vi "DriveExecute_StateSpaceCtrl_1.vi"(8 "error in (no error)":errorcluster) -> (0 "error out":errorcluster)   [LabVIEW 2020]
doc: "Execute for Drie\n\nClosed control loop for drive\n\ninput: \n error in (cluster)\n\noutput:\n error out (cluster)"
uses:
  <vilib>/Rock Robotics/WPI/ThirdParty/Phoenix-LabVIEW/Motor Controller/Controls/CTRE_Phoenix_MotorControl_ControlMode.ctl
  <vilib>/Rock Robotics/WPI/ThirdParty/JAS_Junk/TrajLib/SimpleMotorFF_Calculate.vi
  <vilib>/Rock Robotics/WPI/ThirdParty/JAS_Junk/TrajLib/VI/Util_GetTime_U32.vi
  <vilib>/Rock Robotics/WPI/ThirdParty/JAS_Junk/TrajLib/PIDController_AtSetpoint.vi
  <vilib>/Rock Robotics/WPI/ThirdParty/JAS_Junk/TrajLib/PIDController_SetPIDF.vi
  <vilib>/Rock Robotics/WPI/ThirdParty/JAS_Junk/TrajLib/PIDController_SetDerivativeFilter.vi
  <vilib>/Rock Robotics/WPI/ThirdParty/JAS_Junk/TrajLib/PIDController_SetIntegratorRange.vi
  <vilib>/Rock Robotics/WPI/ThirdParty/JAS_Junk/TrajLib/PIDController_SetTolerancePandV.vi
  <vilib>/Rock Robotics/WPI/ThirdParty/JAS_Junk/TrajLib/PIDController_DisableContinousInput.vi
  <vilib>/Rock Robotics/WPI/ThirdParty/JAS_Junk/TrajLib/PIDController_EnableContinousInput.vi
  <vilib>/Rock Robotics/WPI/ThirdParty/JAS_Junk/TrajLib/PIDController_Reset.vi
  <vilib>/Rock Robotics/WPI/ThirdParty/JAS_Junk/TrajLib/PIDController_New.vi
  <vilib>/Rock Robotics/WPI/ThirdParty/JAS_Junk/TrajLib/PIDController_SetOutputLimits.vi
  <vilib>/Rock Robotics/WPI/ThirdParty/JAS_Junk/TrajLib/SlewRateLimiter_New.vi
  <vilib>/Rock Robotics/WPI/ThirdParty/JAS_Junk/TrajLib/SlewRateLimiter_Reset.vi
  <vilib>/Rock Robotics/WPI/ThirdParty/JAS_Junk/TrajLib/SlewRateLimiter_Calculate.vi
  <vilib>/Rock Robotics/WPI/ThirdParty/JAS_Junk/TrajLib/SlewRateLimiter_SetRate.vi
  <vilib>/Rock Robotics/WPI/ThirdParty/JAS_Junk/TrajLib/PIDController_NewPeriod.vi
  <vilib>/Rock Robotics/SystemInterfaces/NetworkCommunication/NetComm_UsageReport_report.vi
  <vilib>/Rock Robotics/SystemInterfaces/Utilities/FPGA_UtilitiesRead LocalTime.vi
  <vilib>/Rock Robotics/WPI/ThirdParty/JAS_Junk/TrajLib/VI/Util_GetTime_U64.vi
  DriveGlobal.vi
  <vilib>/Rock Robotics/WPI/ThirdParty/Phoenix-LabVIEW/Motor Controller/Get/CTRE_Phoenix_MotorController_GetSelectedSensorData.vi
  <vilib>/Rock Robotics/WPI/ThirdParty/JAS_Junk/TrajLib/Globals/Util_LibraryGlobals.vi
  <vilib>/Rock Robotics/WPI/ThirdParty/JAS_Junk/TrajLib/PIDController_AdvCalculate_FF_Sp_Pv.vi
  <vilib>/Rock Robotics/WPI/ThirdParty/JAS_Junk/TrajLib/Trajectory_Library.lvlib
  <vilib>/Rock Robotics/WPI/ThirdParty/JAS_Junk/TrajLib/Enum/DCMOTOR_TYPES_ENUM.ctl
  <vilib>/Rock Robotics/WPI/ThirdParty/JAS_Junk/TrajLib/Enum/DIFF_DRIVE_ToughBoxMini_GearChoice_ENUM.ctl
  <vilib>/Rock Robotics/Network Tables/NT Write Number.vi
  <vilib>/Rock Robotics/Network Tables/NT Write Boolean.vi
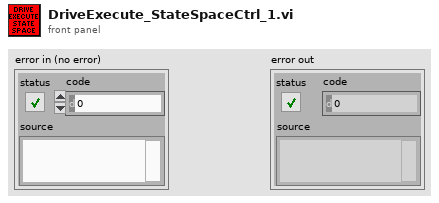
[diagram p1: front panel]
types:
  T1 = typedef "Trajectory_Library.lvlib/DIFF_DRIVE_ToughBoxMini_GearChoice_ENUM.ctl" = enum16{"Ratio_12_75", "Ratio_10_71", "Ratio_8_45", "Ratio_7_31", "Ratio_5_95"}
  T2 = typedef "Trajectory_Library.lvlib/DCMOTOR_TYPES_ENUM.ctl" = enum16{"CIM", "AndyMark 9015", "Andy Mark RS 775 125", "Bag", "BaneBots RS 550", "BaneBots RS 775", "Falcon 500", "Mini CIM", "NEO", "NEO 550", "Romi BuiltIn", "Vex 775 Pro", "Snow Blower AM 2235A", "Bosch Seat AM 3493"}
  T3 = typedef "CTRE_Phoenix_MotorControl_ControlMode.ctl" = u16
  T4 = typedef "WPI_MotorControlDeviceRef.ctl" = cluster{"DeviceStatus":errorcluster, "Type":T5, "PWM":cluster{"PWM Channel":T6, "DeadBand":T7}, "CAN":cluster{"Device Number":u8, "SetOutput VI Ref":variant, "GetOutput VI Ref":variant, "Enable VI Ref":variant, "Disable VI Ref":variant, "Data":variant}, "Invert":bool, "DIO PWM":cluster{"PWM \"Enable\" Channel":T6, "DIOChannel":T8, "PWM Rate":dbl}}
  T5 = typedef "WPI_MotorControlType.ctl" = enum16{"PWM", "CAN", "DIO PWM"}
  T6 = typedef "FPGA_DIOPWMChannel.ctl" = enum8{"PWM 0", "PWM 1", "PWM 2", "PWM 3", "PWM 4", "PWM 5", "PWM 6", "PWM 7", "PWM 8", "PWM 9", "PWM MXP 0", "PWM MXP 1", "PWM MXP 2", "PWM MXP 3", "PWM MXP 4", "PWM MXP 5", "PWM MXP 6", "PWM MXP 7", "PWM MXP 8", "PWM MXP 9", "Invalid"}
  T7 = typedef "WPI_PWMDeadband.ctl" = cluster{"Name":string, "maxPositivePwm":i32, "minPositivePwm":i32, "centerPwm":i32, "maxNegativePwm":i32, "minNegativePwm":i32, "angularRange":u16}
  T8 = typedef "FPGA_DIOChannel.ctl" = enum8{"DIO 0", "DIO 1", "DIO 2", "DIO 3", "DIO 4", "DIO 5", "DIO 6", "DIO 7", "DIO 8", "DIO 9", "DIO MXP 0", "DIO MXP 1", "DIO MXP 2", "DIO MXP 3", "DIO MXP 4", "DIO MXP 5", "DIO MXP 6", "DIO MXP 7", "DIO MXP 8", "DIO MXP 9", "DIO MXP 10", "DIO MXP 11", "DIO MXP 12", "DIO MXP 13", "DIO MXP 14", "DIO MXP 15", "SPI Port CS1", "SPI Port CS2", "SPI Port CS3", "SPI Port MISO", "SPI Port MOSI", "Invalid"}
  T9 = typedef "ADIS16470 Device Reference.ctl" = cluster{"DevStatus":errorcluster, "Hardware Config":T10, "Calibration Complete":refnum<notifier>, "Status Reference":refnum<data-value>, "Data Reference":refnum<data-value>, "Sychronous Process VI":T13, "Cmd FIFO":refnum<k33>, "Source":T14, "Data FIFO":refnum<k33>, "Calibration Time (ms)":u32, "Data Reference":refnum<data-value>}
  T10 = typedef "ADIS16470 Hardware Configuration.ctl" = cluster{"SPI Clock Rate (Hz)":dbl, "IMU SPI Mode (3)":T11, "IMU Reset Pin":T8, "IMU SPI Bus":T12, "IMU Data Ready Pin":T8, "Stall Config":cluster{"Pow2BytesPerRead":u8, "StallTicks":u16, "CsToSclkTicks":u8}}
  T11 = typedef "WPI_SPIMode.ctl" = enum16{"Mode 0 (Clk Idle Low,Sample on Leading)", "Mode 1 (Clk Idle Low,Sample on Trailing)", "Mode 2 (Clk Idle High,Sample on Leading)", "Mode 3 (Clk Idle High,Sample on Trailing)"}
  T12 = typedef "spi_bus.ctl" = enum16{"SPI On-Board, CS0", "SPI On-Board, CS1", "SPI On-Board, CS2", "SPI On-Board, CS3", "SPI MXP", "Invalid"}
  T13 = typedef "ADIS16470 Process.ctl" = refnum<vi>
  T14 = typedef "FPGA_CounterEncoderSourceConvertionLVSourceType.ctl" = cluster{"DevStatus":errorcluster, "AnalogTriggerMode?":bool, "DigitalMode":cluster{"DIO Channel":T15}, "AnalogTriggerMode":cluster{"AnalogTriggerIndex":T16, "OutputType":T17}}
  T15 = typedef "FPGA_DIODigitalSourceChannel.ctl" = enum8{"DIO 0", "DIO 1", "DIO 2", "DIO 3", "DIO 4", "DIO 5", "DIO 6", "DIO 7", "DIO 8", "DIO 9", "DIO MXP 0", "DIO MXP 1", "DIO MXP 2", "DIO MXP 3", "DIO MXP 4", "DIO MXP 5", "DIO MXP 6", "DIO MXP 7", "DIO MXP 8", "DIO MXP 9", "DIO MXP 10", "DIO MXP 11", "DIO MXP 12", "DIO MXP 13", "DIO MXP 14", "DIO MXP 15", "SPI Port CS1", "SPI Port CS2", "SPI Port CS3", "SPI Port MISO", "SPI Port MOSI", "Disabled"}
  T16 = typedef "FPGA_AnalogTriggerIndex.ctl" = enum8{"Trig 0", "Trig 1", "Trig 2", "Trig 3", "Trig 4", "Trig 5", "Trig 6", "Trig 7", "Invalid"}
  T17 = typedef "FPGA_AnalogTriggerOutType.ctl" = enum16{"InWindow", "TriggerState", "Rising", "Falling"}
  T18 = typedef "ADIS16470 Data.ctl" = cluster{"XAngle":dbl, "YAngle":dbl, "ZAngle":dbl}
  T19 = typedef "Trajectory_Library.lvlib/LINEAR_SYSTEM.ctl" = cluster{"m_A":T20, "m_B":T20, "m_C":T20, "m_D":T20, "States":i32, "Inputs":i32, "Outputs":i32}
  T20 = typedef "NI_Matrix.lvlib/RealMatrix.ctl" = dbl[][]
  T21 = typedef "Trajectory_Library.lvlib/LINEAR_SYSTEM_LOOP_DIFF_DRV_CTRL_PARAMS.CTL" = cluster{"Left Vel Model Std Dev m/s":dbl, "Left Vel Meas Std Dev m/s":dbl, "Left Vel Ctrl Tol m/s":dbl, "Max Control Effort":dbl, "Right Vel Ctrl Tol m/s":dbl, "Right Vel Meas Std Dev m/s":dbl, "Right Vel Model Std Dev m/s":dbl}
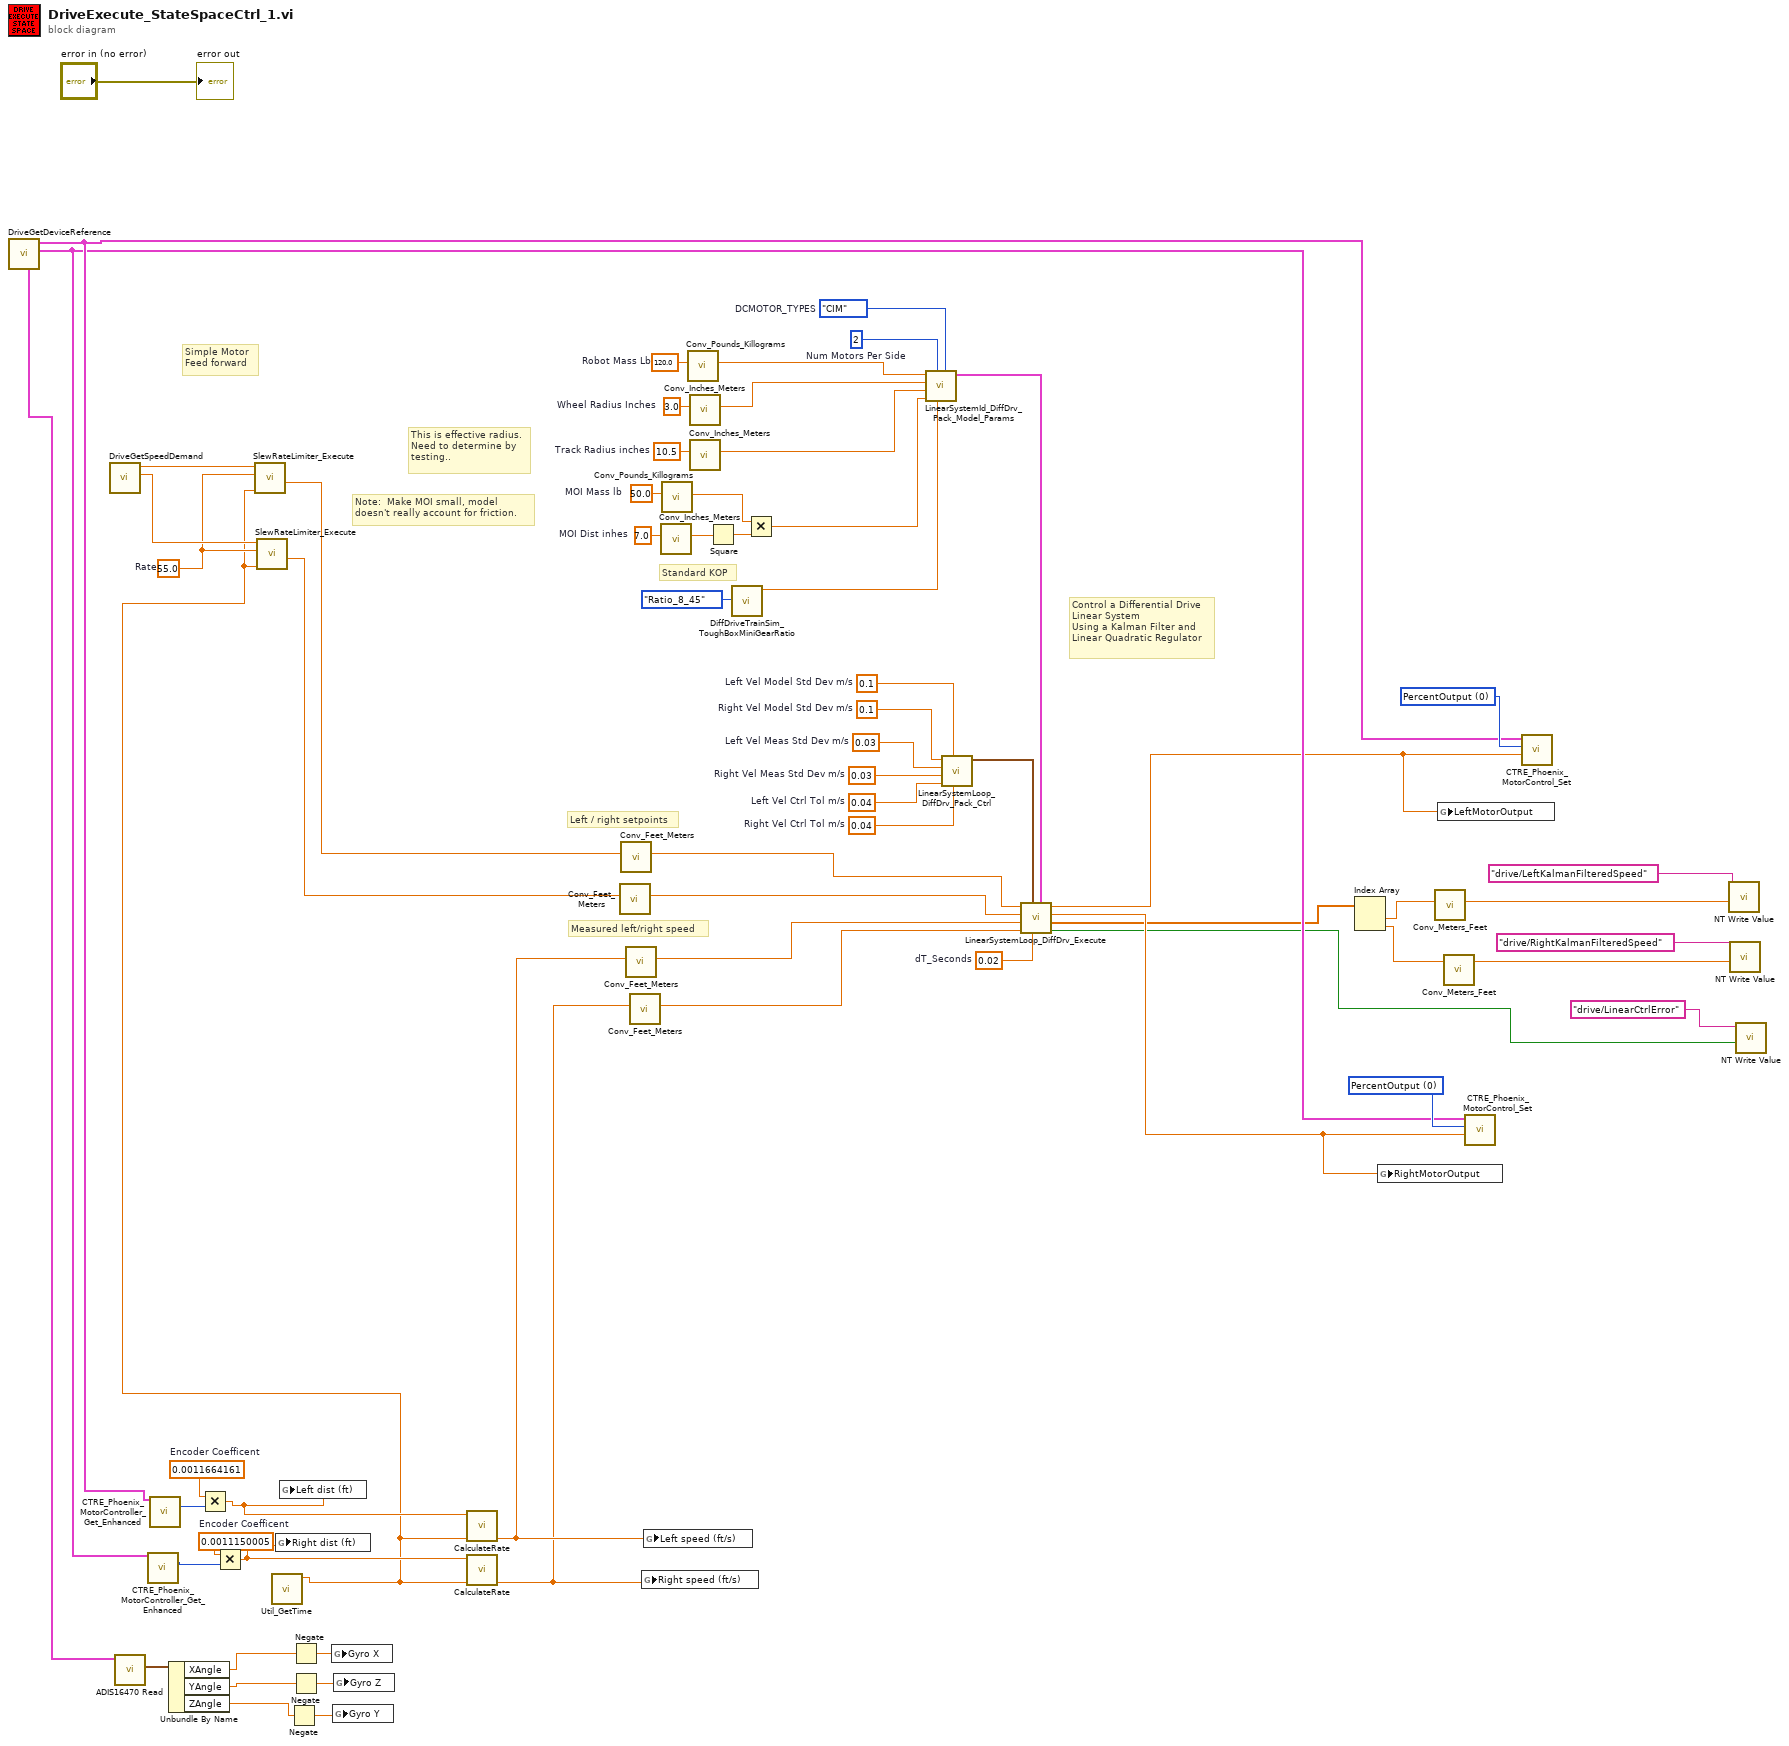
[diagram p0: block diagram]
diagram:
  w12 = 0.02  # dT_Seconds
  w16 = 10.5  # Track Radius inches
  w23 = 7.0  # MOI Dist inhes
  w24 = 50.0  # MOI Mass lb
  w26 = 3.0  # Wheel Radius Inches
  w28 = 120.0  # Robot Mass Lb
  w37 = 0.1  # Right Vel Model Std Dev m/s
  w38 = 0.03  # Left Vel Meas Std Dev m/s
  w39 = 0.03  # Right Vel Meas Std Dev m/s
  w40 = 0.04  # Left Vel Ctrl Tol m/s
  w41 = 0.1  # Left Vel Model Std Dev m/s
  w42 = 0.04  # Right Vel Ctrl Tol m/s
  w43 = 2  # Num Motors Per Side
  w44 = DCMOTOR_TYPES_ENUM."CIM"  # DCMOTOR_TYPES
  w11 = 55.0  # Rate
  w57 = 0.0011150005  # Encoder Coefficent
  w59 = 0.0011664161  # Encoder Coefficent
  w66 = T3 0 items=["PercentOutput"=0, "Position"=1, "Velocity"=2, "Current"=3, "Follower"=5, "MotionProfile"=6, "MotionMagic"=7, "MotionProfileArc"=10, "Disabled"=15] ("Control Mode")
  w67 = T3 0 items=["PercentOutput"=0, "Position"=1, "Velocity"=2, "Current"=3, "Follower"=5, "MotionProfile"=6, "MotionMagic"=7, "MotionProfileArc"=10, "Disabled"=15] ("Control Mode")
  # "Standard KOP"
  # "This is effective radius.\nNeed to determine by\ntesting.."
  # "Note:  Make MOI small, model\ndoesn't really account for friction."
  # "Measured left/right speed"
  # "Left / right setpoints"
  # "Control a Differential Drive\nLinear System\nUsing a Kalman Filter and \nLinear Quadratic Regulator"
  # "Simple Motor\nFeed forward"
  n1 = call "DriveGetDeviceReference.vi"() -> ("RightDriveTrain"=w61:T4, "LeftDriveTrain"=w62:T4, "Gryo"=w63:T9)  [unwired: 9 in]
  n2 = call "DriveGetSpeedDemand.vi"() -> ("RSpeedDemand (ft/s)"=w53:dbl, "LSpeedDemand (ft/s)"=w54:dbl)  [unwired: 10 in]
  n3 = call <vilib>:"ADIS16470 Read.vi"("ADIS16470DevRef"=w63) -> ("ADIS16470 Value"=w64:T18)  [unwired: 7 in, 3 out]
  n4 = call-poly <vilib>:"CTRE_Phoenix_MotorController_Get_Enhanced.vi"("PhoenixMotorControlDevRef"=w61) -> ("Position (Raw Sensor Units)"=w56:i32)  [unwired: 11 in, 3 out]
  n5 = call-poly <vilib>:"CTRE_Phoenix_MotorController_Get_Enhanced.vi"("PhoenixMotorControlDevRef"=w62) -> ("Position (Raw Sensor Units)"=w60:i32)  [unwired: 11 in, 3 out]
  n6 = Unbundle By Name(w64) -> ("XAngle"=w47:dbl, "YAngle"=w49:dbl, "ZAngle"=w48:dbl)
  n7 = Multiply(x=w59, y=w60) -> (x*y=w58:dbl)
  n8 = Multiply(x=w57, y=w56) -> (x*y=w55:dbl)
  n9 = call <vilib>:"Util_GetTime.vi"() -> ("FPGA_Time_Seconds"=w10:dbl)  [unwired: 9 in, 2 out]
  n10 = call <vilib>:"SlewRateLimiter_Execute.vi"("Time"=w10, "PositiveRate"=w11, "Input"=w54) -> ("Output"=w36:dbl)  [unwired: 7 in, 1 out]
  n11 = call <vilib>:"SlewRateLimiter_Execute.vi"("Time"=w10, "PositiveRate"=w11, "Input"=w53) -> ("Output"=w35:dbl)  [unwired: 7 in, 1 out]
  n12 = global write "DriveGlobal.vi" "Right dist (ft)"(w55) -> ()
  n13 = global write "DriveGlobal.vi" "Left dist (ft)"(w58) -> ()
  n14 = Negate(x=w48) -> (-x=w51:dbl)
  n15 = Negate(x=w47) -> (-x=w52:dbl)
  n16 = Negate(x=w49) -> (-x=w50:dbl)
  n17 = global write "DriveGlobal.vi" "Gyro X"(w52) -> ()
  n18 = global write "DriveGlobal.vi" "Gyro Y"(w51) -> ()
  n19 = global write "DriveGlobal.vi" "Gyro Z"(w50) -> ()
  n20 = call "CalculateRate.vi"("Time (s)"=w10, "Distance (units)"=w58) -> ("Rate (units/s)"=w32:dbl)  [unwired: 9 in]
  n21 = call "CalculateRate.vi"("Time (s)"=w10, "Distance (units)"=w55) -> ("Rate (units/s)"=w31:dbl)  [unwired: 9 in]
  n22 = call <vilib>:"Conv_Feet_Meters.vi"("Feet"=w35) -> ("Meters"=w33:dbl)  [unwired: 10 in]
  n23 = call <vilib>:"Conv_Feet_Meters.vi"("Feet"=w36) -> ("Meters"=w34:dbl)  [unwired: 10 in]
  n24 = call <vilib>:"Conv_Feet_Meters.vi"("Feet"=w32) -> ("Meters"=w30:dbl)  [unwired: 10 in]
  n25 = call <vilib>:"Conv_Feet_Meters.vi"("Feet"=w31) -> ("Meters"=w29:dbl)  [unwired: 10 in]
  n26 = global write "DriveGlobal.vi" "Right speed (ft/s)"(w31) -> ()
  n27 = global write "DriveGlobal.vi" "Left speed (ft/s)"(w32) -> ()
  n28 = call <vilib>:"Conv_Inches_Meters.vi"("INCH"=w23) -> ("Meters"=w22:dbl)  [unwired: 10 in]
  n29 = call <vilib>:"Conv_Pounds_Killograms.vi"("Pounds"=w24) -> ("Killograms"=w20:dbl)  [unwired: 10 in]
  n30 = call <vilib>:"Conv_Pounds_Killograms.vi"("Pounds"=w28) -> ("Killograms"=w27:dbl)  [unwired: 10 in]
  n31 = call <vilib>:"Conv_Inches_Meters.vi"("INCH"=w26) -> ("Meters"=w25:dbl)  [unwired: 10 in]
  n32 = call <vilib>:"Conv_Inches_Meters.vi"("INCH"=w16) -> ("Meters"=w15:dbl)  [unwired: 10 in]
  n33 = Square(x=w22) -> (x^2=w21:dbl)
  n34 = call <vilib>:"DiffDriveTrainSim_ToughBoxMiniGearRatio.vi"("ToughBoxMiniGear"=DIFF_DRIVE_ToughBoxMini_GearChoice_ENUM."Ratio_8_45") -> ("GearRatio"=w17:dbl)  [unwired: 10 in]
  n35 = Multiply(x=w20, y=w21) -> (x*y=w19:dbl)
  n36 = call <vilib>:"LinearSystemId_DiffDrv_Pack_Model_Params.vi"("DCMOTOR_TYPES"=w44, "Gear Ratio"=w17, "Num Motors Per Side"=w43, "MOI-KgM2"=w19, "Track Radius-m"=w15, "Wheel Radius-M"=w25, "Mass-Kg"=w27) -> ("DiffDrv_LinearSystem"=w45:T19)  [unwired: 4 in]
  n37 = call <vilib>:"LinearSystemLoop_DiffDrv_Pack_Ctrl.vi"("Right Vel Ctrl Tol m/s"=w42, "Left Vel Model Std Dev m/s"=w41, "Left Vel Ctrl Tol m/s"=w40, "Right Vel Meas Std Dev m/s"=w39, "Left Vel Meas Std Dev m/s"=w38, "Right Vel Model Std Dev m/s"=w37) -> ("LinearSystemLoop_DiffDrv_Ctrl_Params"=w46:T21)  [unwired: 5 in]
  n38 = call <vilib>:"LinearSystemLoop_DiffDrv_Execute.vi"("Linear System"=w45, "dT_Seconds"=w12, "LinearSystemLoop_DiffDrv_Control_Params"=w46, "Right Vel PV m/s"=w29, "Left Vel PV m/s"=w30, "Right Vel SP m/s"=w33, "Left Vel SP m/s"=w34) -> ("Error"=w1:bool, "Filtered States"=w9:dbl[], "Right Motor Dmd"=w13:dbl, "Left Motor Dmd"=w14:dbl)  [unwired: 1 out]
  n39 = Index Array(array=w9) -> (element #1=w8:dbl, element #2=w7:dbl)  [unwired: 2 in]
  n40 = global write "DriveGlobal.vi" "RightMotorOutput"(w13) -> ()
  n41 = call <vilib>:"Conv_Meters_Feet.vi"("Meters"=w8) -> ("Feet"=w6:dbl)  [unwired: 10 in]
  n42 = global write "DriveGlobal.vi" "LeftMotorOutput"(w14) -> ()
  n43 = call <vilib>:"Conv_Meters_Feet.vi"("Meters"=w7) -> ("Feet"=w5:dbl)  [unwired: 10 in]
  n44 = call <vilib>:"CTRE_Phoenix_MotorControl_Set.vi"("Output"=w13, "Control Mode"=w66, "PhoenixMotorControlDevRef"=w61) -> ()  [unwired: 7 in, 2 out]
  n45 = call <vilib>:"CTRE_Phoenix_MotorControl_Set.vi"("Output"=w14, "Control Mode"=w67, "PhoenixMotorControlDevRef"=w62) -> ()  [unwired: 7 in, 2 out]
  n46 = call-poly <vilib>:"NT Write Value.vi"("value"=w6, "name"="drive/LeftKalmanFilteredSpeed") -> ()  [unwired: 9 in, 1 out]
  n47 = call-poly <vilib>:"NT Write Value.vi"("value"=w5, "name"="drive/RightKalmanFilteredSpeed") -> ()  [unwired: 9 in, 1 out]
  n48 = call-poly <vilib>:"NT Write Value.vi"("value"=w1, "name"="drive/LinearCtrlError") -> ()  [unwired: 9 in, 1 out]
  "error out" <- "error in (no error)"
